vi "libssh2_session_handshake_tcp - invalid session - no error 1097.vi"() -> ()   [LabVIEW 2013, in "libssh2_tests.lvlib"]
uses:
  libssh2_tests.lvlib
  libssh2/Session Refnum.ctl
  libssh2/libssh2_init_default.vi
  <vilib>/Utility/error.llb/General Error Handler.vi
  <vilib>/addons/_JKI Toolkits/Caraya/classes/Assert/Assert.vi
  <vilib>/addons/_JKI Toolkits/Caraya/classes/Assert/Assert Not Error.vi
  <vilib>/addons/_JKI Toolkits/Caraya/classes/Test/Test.lvclass
  libssh2/libssh2.lvlib
panel:
  out "error out":errorcluster
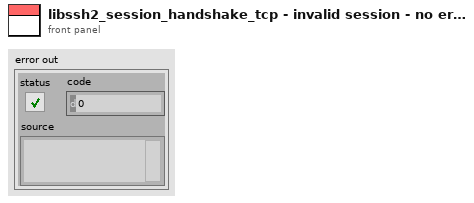
[diagram p1: front panel]
types:
  T1 = typedef "libssh2.lvlib/Session Refnum.ctl" = refnum<k1>
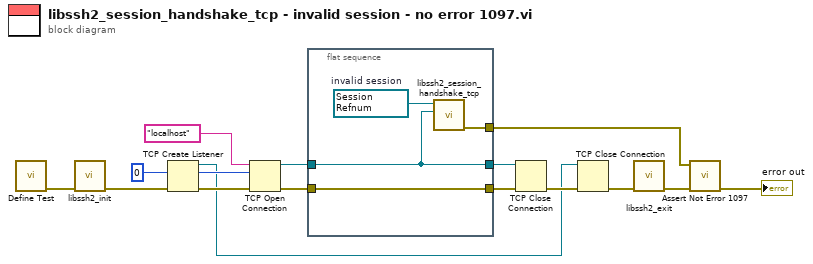
[diagram p0: block diagram]
diagram:
  n1 = call <vilib>:"Define Test.vi"() -> ("error out"=w15:errorcluster)  [unwired: 10 in, 1 out]
  n2 = call-poly "libssh2_init.vi"("error in (no error)"=w15) -> ("error out"=w12:errorcluster)  [unwired: 10 in]
  n3 = TCP Create Listener(8:w12, 10:u16 0 ("remote port or service name")) -> (0:w11:errorcluster, 2:w8:u16, 3:w4:refnum<k5>)  [unwired: 3 in]
  n4 = TCP Open Connection(address="localhost", remote port or service name=w8, error in (no error)=w11) -> (connection ID=w2:refnum<k5>, error out=w1:errorcluster)  [unwired: 2 in]
  n5 = flat-sequence {
    tunnel: [w19] -> w13
    tunnel: w1 -> [w19]
    tunnel: [w18] -> w3
    tunnel: w2 -> [w17]
    tunnel: [w17] -> w7
    frame #0 {
      w20 = T1 refnum items=["Session"]  # invalid session
      n6 = call "libssh2_session_handshake_tcp.vi"("tcp connection"=w17, "session"=w20) -> ("error out"=w18:errorcluster)  [unwired: 9 in]
    }
  }
  n7 = TCP Close Connection(connection ID=w7, error in (no error)=w13) -> (error out=w6:errorcluster)  [unwired: 1 in, 1 out]
  n8 = TCP Close Connection(connection ID=w4, error in (no error)=w6) -> (error out=w5:errorcluster)  [unwired: 1 in, 1 out]
  n9 = call "libssh2_exit.vi"("error in (no error)"=w5) -> ("error out"=w14:errorcluster)  [unwired: 10 in]
  n10 = call "Assert Not Error 1097.vi"("error in (no error)"=w14, "actual value"=w3) -> ("error out"=→"error out":errorcluster)  [unwired: 9 in]
